vi "Testing.vi"() -> ()   [LabVIEW 2025]
uses:
  <vilib>/Mines/ME-DAQ/InputDAQ/MEGN300InputDAQ/MultipleChannelOneSample.vi
panel:
  in  "stop":bool
  out "data out":string
  out "data":dbl[](array[numeric]) format="%0.2f"
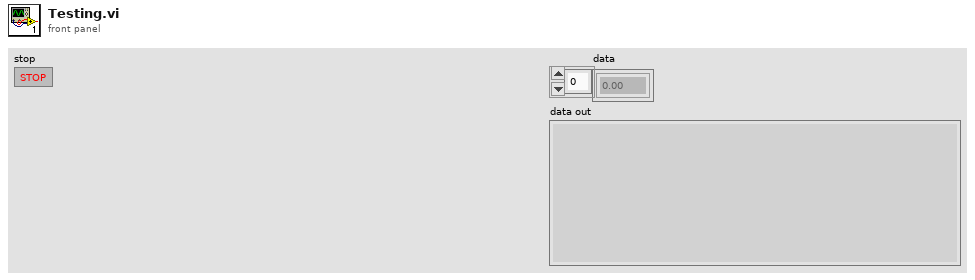
[diagram p1: front panel]
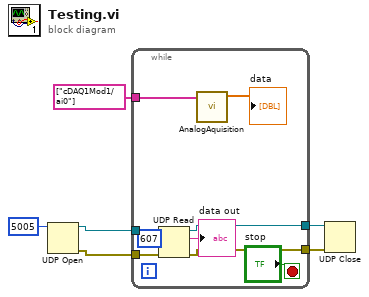
[diagram p0: block diagram]
diagram:
  n1 = UDP Open(11:u16 5005 ("port")) -> (port=w5:refnum<k16>, 0:w3:errorcluster)  [unwired: 4 in, 1 out]
  n2 = while {
    tunnel: tag[] ["cDAQ1Mod1/ai0"] ("DAQmx Physical Channels") -> [w15]
    tunnel: w5 -> [w13]
    tunnel: [w12] -> w4
    tunnel: w3 -> [w11]
    tunnel: [w10] -> w2
    stop <- "stop" stop-if-true
    n3 = UDP Read(connection ID=w13, max size (548)=607, 8:w11) -> (data out=→"data out":string, error out=w10:errorcluster, 3:w12:refnum<k16>)  [unwired: 1 in, 2 out]
    n4 = call-poly <vilib>:"AnalogAquisition.vi"("DAQmx Physical Channels"=w15) -> ("data"=→"data":dbl[])  [unwired: 9 in, 1 out]
  }
  n5 = UDP Close(connection ID=w4, 8:w2) -> ()  [unwired: 2 out]
